vi "MakeTurn.vi"(8 "error in (no error)":errorcluster, 11 "Game in":refnum<class "Game.lvclass">) -> (0 "error out":errorcluster, 1 "GameResult":T2, 2 "Finished?":bool, 3 "Game out":refnum<class "Game.lvclass">)   [LabVIEW 2015, in "TronviewGame.lvlib" / "Game.lvclass"]
uses:
  Game.lvclass
  GameResult.ctl
  TronVIEWBotAPI/BotData.ctl
  TronVIEWBotAPI/MatchState.ctl
  Game.lvclass/Game.ctl
  Board/Board.lvclass
  TronVIEWBotAPI/TronVIEWBotAPI.lvlib
panel:
  in  "BotData":T1
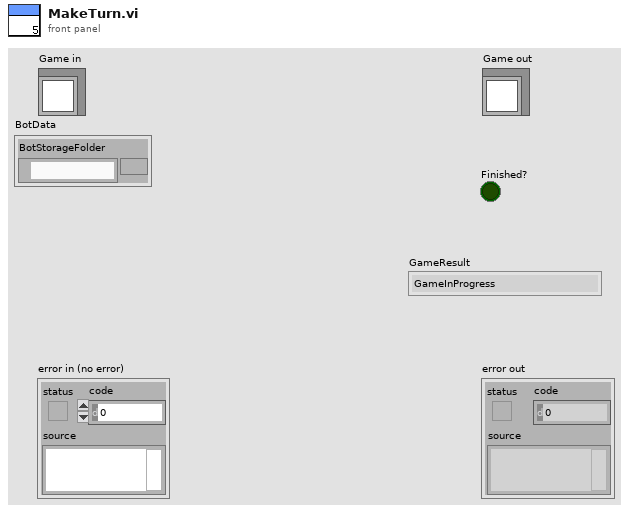
[diagram p1: front panel]
types:
  T1 = typedef "TronVIEWBotAPI.lvlib/BotData.ctl" = cluster{"BotStorageFolder":path}
  T2 = typedef "TronviewGame.lvlib/Game.lvclass/GameResult.ctl" = enum16{"GameInProgress", "Draw", "Player1Won", "Player2Won"}
  T3 = typedef "TronVIEWBotAPI.lvlib/MatchState.ctl" = cluster{"OpponentName":string, "PlayerScore":u32, "OpponentScore":u32}
  T4 = typedef "TronVIEWBotAPI.lvlib/GameState.ctl" = cluster{"CurrentBotPosition":T5, "Board":bool[][], "CurrentOpponentPosition":T5}
  T5 = typedef "TronviewGame.lvlib/Board.lvclass/Position.ctl" = cluster{"Column":i32, "Row":i32}
  T6 = typedef "TronVIEWBotAPI.lvlib/BotVIRefnum.ctl" = refnum<vi>
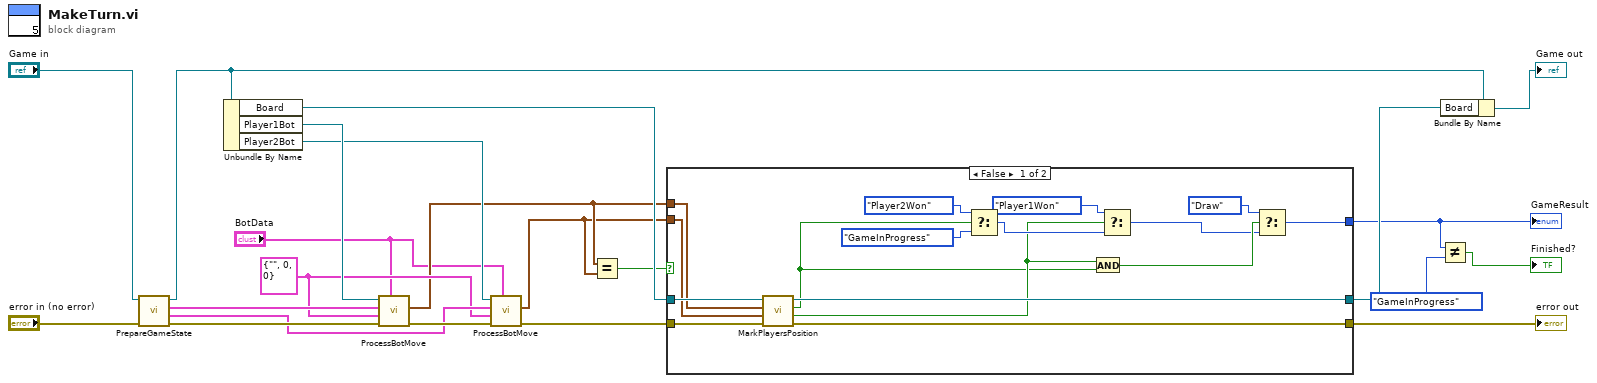
[diagram p0: block diagram]
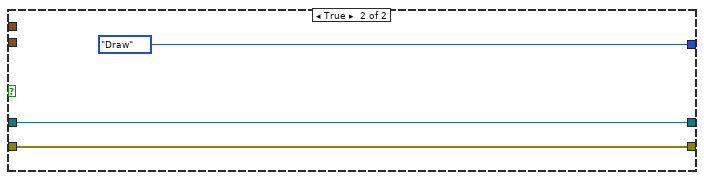
[diagram p2: hidden frame]
diagram:
  w4 = T3 {"OpponentName"="", "PlayerScore"=0, "OpponentScore"=0} ("MatchState")
  n1 = call "PrepareGameState.vi"("error in (no error)"="error in (no error)", "Game in"="Game in") -> ("error out"=w10:errorcluster, "Bot2GameState"=w5:T4, "Bot1GameState"=w6:T4, "Game out"=w11:refnum<class "Game.lvclass">)  [unwired: 6 in]
  n2 = Unbundle By Name(w11) -> ("Board"=w18:refnum<class "Board.lvclass">, "Player1Bot"=w21:T6, "Player2Bot"=w20:T6)
  n3 = call "ProcessBotMove.vi"("BotData"="BotData", "error in (no error)"=w10, "MatchState"=w4, "GameState"=w6, "Bot in"=w21) -> ("error out"=w19:errorcluster, "NewPlayerPosition"=w3:T5)  [unwired: 4 in, 1 out]
  n4 = call "ProcessBotMove.vi"("BotData"="BotData", "error in (no error)"=w19, "MatchState"=w4, "GameState"=w5, "Bot in"=w20) -> ("error out"=w16:errorcluster, "NewPlayerPosition"=w2:T5)  [unwired: 4 in, 1 out]
  n5 = Equal?(x=w3, y=w2) -> (x = y?=w14:bool)
  n6 = case shown="False" w14 {
    tunnel: w18 -> [w38 w41]
    tunnel: [w37 w41] -> w17
    tunnel: w16 -> [w36 w40]
    tunnel: [w35 w40] -> w15
    tunnel: w2 -> [w25 _]
    tunnel: w3 -> [w34 _]
    tunnel: [w32 GameResult."Draw" ("GameResult")] -> w9
    frame False {
      n7 = call "MarkPlayersPosition.vi"("error in (no error)"=w36, "Player2NewPosition"=w25, "Player1NewPosition"=w34, "Board in"=w38) -> ("error out"=w35:errorcluster, "Player2AlreadyOccupied"=w24:bool, "Player1AlreadyOccupied"=w23:bool, "Board out"=w37:refnum<class "Board.lvclass">)  [unwired: 4 in]
      n8 = Select(t=GameResult."Player2Won", s=w23, f=GameResult."GameInProgress" ("GameResult")) -> (s? t:f=w29:T2)
      n9 = And(x=w24, y=w23) -> (x .and. y?=w33:bool)
      n10 = Select(t=GameResult."Player1Won", s=w24, f=w29) -> (s? t:f=w27:T2)
      n11 = Select(t=GameResult."Draw", s=w33, f=w27) -> (s? t:f=w32:T2)
    }
    frame True {
    }
  }
  "error out" <- w15
  "GameResult" <- w9
  n12 = Not Equal?(x=w9, y=GameResult."GameInProgress") -> (x != y?=→"Finished?":bool)
  n13 = Bundle By Name(cluster=w11, "Board"=w17) -> (→"Game out":refnum<class "Game.lvclass">)
